vi "Lookup MIME Type.vi"(8 "error in (no error)":errorcluster, 10 "Path":path) -> (0 "error out":errorcluster, 2 "MIME Type":string)   [LabVIEW 2023, in "Server.lvclass"]
uses:
  Server.lvclass
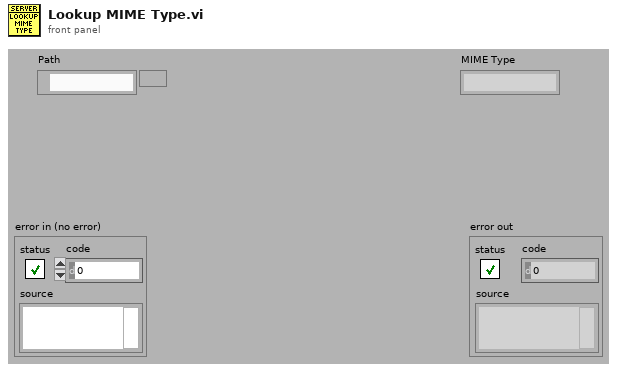
[diagram p1: front panel]
types:
  T1 = typedef "Server.lvclass/ObjectAttributes.ctl" = cluster{"Static Data":path, "MIME Types":variant, "Shutdown":bool, "API Queue":refnum<queue>, "ControlEndpoints":map{string, cluster{"Ref":refnum<vi>, "Mode":T2}}, "EventEndpoints":map{string, refnum<user-event>}}
  T2 = typedef "Server.lvclass/Control Ref Endpoint Access Mode.ctl" = enum16{"None", "Read/Write", "Read Only", "Write Only"}
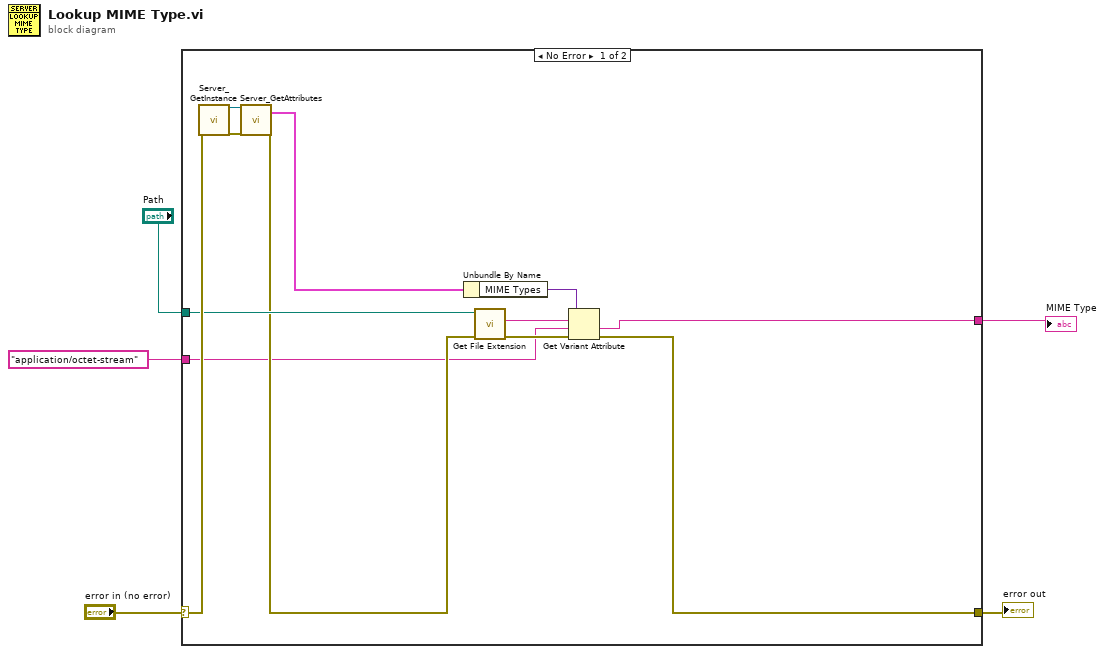
[diagram p0: block diagram]
diagram:
  n1 = case shown="No Error" "error in (no error)" {
    selector: "error in (no error)" -> [w16 w19]
    tunnel: [w7 w19] -> w4
    tunnel: [w10 w18] -> w3
    tunnel: "Path" -> [w9 _]
    tunnel: "application/octet-stream" -> [w6 w18]
    frame No Error {
      n2 = call "Server_GetInstance.vi"("error in (no error)"=w16) -> ("reference out"=w17:refnum<class "Server.lvclass">, "error out"=w15:errorcluster)  [unwired: 14 in, 3 out]
      n3 = call "Server_GetAttributes.vi"("reference in"=w17, "error in (no error)"=w15) -> ("Data"=w11:T1, "error out"=w8:errorcluster)  [unwired: 14 in, 2 out]
      n4 = Unbundle By Name(w11) -> ("MIME Types"=w13:variant)
      n5 = call <vilib>:"Get File Extension.vi"("error in (no error)"=w8, "file"=w9) -> ("error out"=w14:errorcluster, "lowercase file extension"=w12:string)  [unwired: 5 in, 3 out]
      n6 = Get Variant Attribute(Variant=w13, name=w12, default value (empty Variant)=w6, error in=w14) -> (value=w10:string, error out=w7:errorcluster)  [unwired: 2 out]
    }
    frame Error {
    }
  }
  "error out" <- w4
  "MIME Type" <- w3
